vi "SavePhasor.vi"(0 "Intensity":dbl[][](array[numeric]), 1 "G Data":dbl[][](array[numeric]), 2 "S Data":dbl[][](array[numeric]), 3 "Threshold (max)":dbl=0.0035, 4 "Threshold (min)":dbl=0.002, 5 "Auto Scale?":bool=TRUE, 6 "Phasor Grids":i32, 7 "error in":errorcluster, 8 "G_max":dbl=1.1, 9 "Index Name":string, 10 "G_min":dbl=-0.1, 12 "S_max":dbl=1.1, 13 "Enable?":bool, 14 "S_min":dbl=-0.1, 15 "Time Stamp?":bool, 16 "path":path, 17 "Experiment Name":string, 18 "File Name":string, 19 "Identify Name":string, 26 "Crop Pixels":u16=40) -> (21 "img cancelled":bool, 27 "error out":errorcluster)   [LabVIEW 2018]
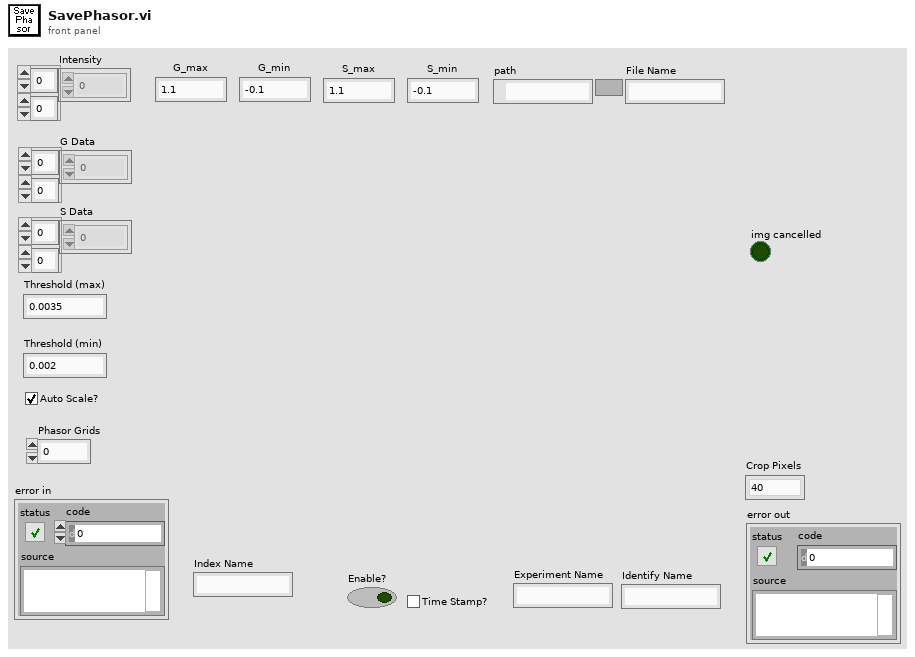
[diagram p1: front panel]
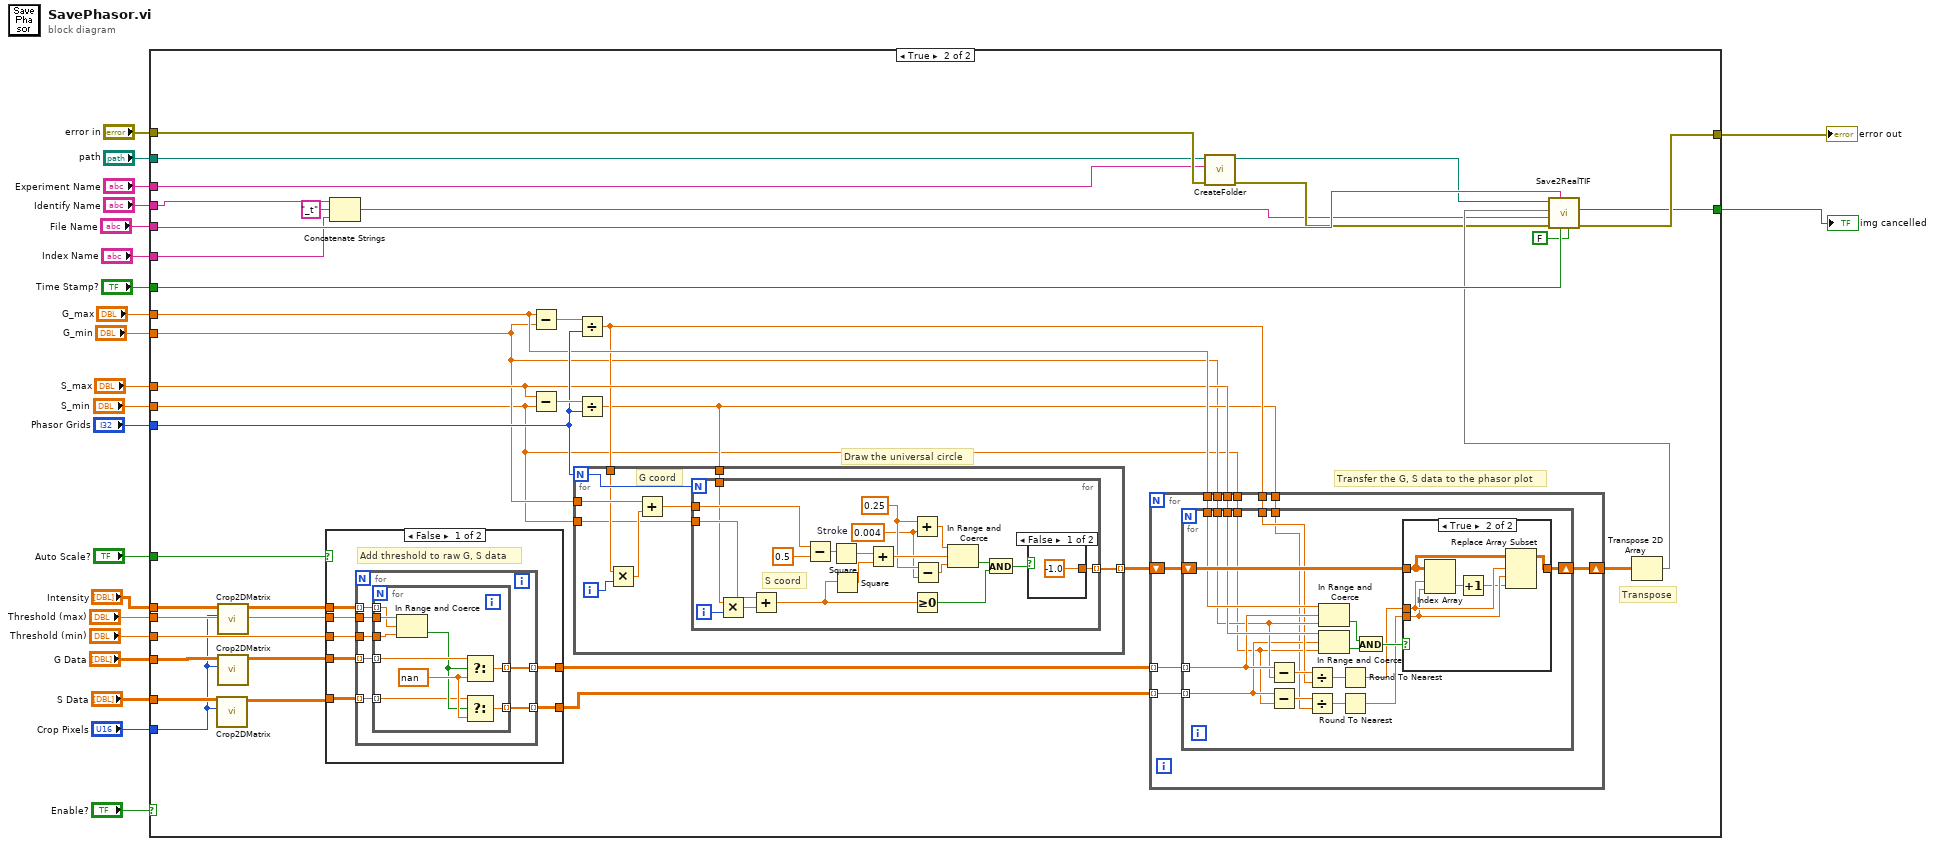
[diagram p0: block diagram]
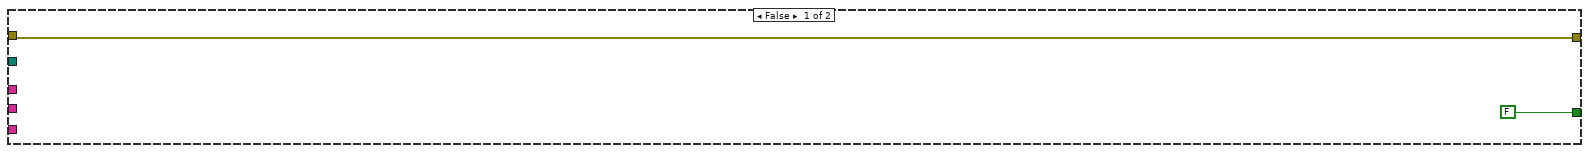
[diagram p2: hidden frame]
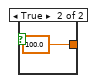
[diagram p5: hidden frame]
diagram:
  n1 = case shown="True" "Enable?" {
    tunnel: "S Data" -> [_ w37]
    tunnel: "G Data" -> [_ w38]
    tunnel: "Threshold (min)" -> [_ w59]
    tunnel: "Threshold (max)" -> [_ w58]
    tunnel: "Auto Scale?" -> [_ w57]
    tunnel: "Intensity" -> [_ w41]
    tunnel: "Phasor Grids" -> [_ w54]
    tunnel: "G_max" -> [_ w53]
    tunnel: "S_max" -> [_ w52]
    tunnel: "G_min" -> [_ w49]
    tunnel: "S_min" -> [_ w48]
    tunnel: [w24 w47] -> w11
    tunnel: "error in" -> [w24 w34]
    tunnel: [FALSE ("save cancelled") w46] -> w8
    tunnel: "path" -> [_ w33]
    tunnel: "Experiment Name" -> [_ w32]
    tunnel: "Identify Name" -> [_ w27]
    tunnel: "File Name" -> [_ w45]
    tunnel: "Time Stamp?" -> [_ w44]
    tunnel: "Crop Pixels" -> [_ w35]
    tunnel: "Index Name" -> [_ w26]
    frame False {
    }
    frame True {
      # "Transpose"
      # "Transfer the G, S data to the phasor plot"
      # "Draw the universal circle"
      n2 = call "Crop2DMatrix.vi"("Crop Pixels"=w35, "Data"=w37) -> ("Cropped Data"=w36:dbl[][])  [unwired: 9 in]
      n3 = call "Crop2DMatrix.vi"("Crop Pixels"=w35, "Data"=w41) -> ("Cropped Data"=w40:dbl[][])  [unwired: 9 in]
      n4 = call "Crop2DMatrix.vi"("Crop Pixels"=w35, "Data"=w38) -> ("Cropped Data"=w39:dbl[][])  [unwired: 9 in]
      n5 = case shown="False" w57 {
        tunnel: w40 -> [w69 _]
        tunnel: w58 -> [w68 _]
        tunnel: w59 -> [w67 _]
        tunnel: w39 -> [w66 w87]
        tunnel: w36 -> [w65 w86]
        tunnel: [w64 w87] -> w61
        tunnel: [w63 w86] -> w60
        frame False {
          # "Add threshold to raw G, S data"
          n6 = for {
            tunnel: w69 -> [w76] mode=indexing
            tunnel: w68 -> [w75]
            tunnel: [w74] -> w64 mode=indexing
            tunnel: w67 -> [w73]
            tunnel: w66 -> [w72] mode=indexing
            tunnel: w65 -> [w71] mode=indexing
            tunnel: [w70] -> w63 mode=indexing
            n7 = for {
              tunnel: w76 -> [w82] mode=indexing
              tunnel: w75 -> [w84]
              tunnel: [w85] -> w74 mode=indexing
              tunnel: w73 -> [w83]
              tunnel: w72 -> [w81] mode=indexing
              tunnel: w71 -> [w78] mode=indexing
              tunnel: [w77] -> w70 mode=indexing
              w80 = nan ("f")
              n8 = In Range and Coerce(upper limit=w84, x=w82, lower limit=w83) -> (In Range?=w79:bool)  [unwired: 1 out]
              n9 = Select(t=w81, s=w79, f=w80) -> (s? t:f=w85:dbl)
              n10 = Select(t=w78, s=w79, f=w80) -> (s? t:f=w77:dbl)
            }
          }
        }
        frame True {
        }
      }
      n11 = Concatenate Strings(w27, "_t" ("string"), w26) -> (w25:string)
      n12 = Subtract(x=w53, y=w49) -> (x-y=w56:dbl)
      n13 = Subtract(x=w52, y=w48) -> (x-y=w55:dbl)
      n14 = Divide(x=w56, y=w54) -> (x/y=w51:dbl)
      n15 = Divide(x=w55, y=w54) -> (x/y=w50:dbl)
      n16 = for {
        N: w54 -> [w132]
        tunnel: [w131] -> w62 mode=indexing
        tunnel: w49 -> [w130]
        tunnel: w51 -> [w127]
        tunnel: w48 -> [w125]
        tunnel: w50 -> [w124]
        i -> [w129]
        # "G coord"
        n17 = Multiply(x=w127, y=w129) -> (x*y=w128:dbl)
        n18 = Add(x=w130, y=w128) -> (x+y=w126:dbl)
        n19 = for {
          N: w132 -> [_]
          tunnel: w126 -> [w151]
          tunnel: [w144] -> w131 mode=indexing
          tunnel: w125 -> [w143]
          tunnel: w124 -> [w141]
          i -> [w142]
          w137 = 0.004  # Stroke
          w138 = 0.25 ("x")
          # "S coord"
          n20 = Multiply(x=w141, y=w142) -> (x*y=w140:dbl)
          n21 = Add(x=w143, y=w140) -> (x+y=w136:dbl)
          n22 = Subtract(x=w151, y=0.5) -> (x-y=w150:dbl)
          n23 = Square(x=w150) -> (x^2=w149:dbl)
          n24 = Square(x=w136) -> (x^2=w148:dbl)
          n25 = Add(x=w149, y=w148) -> (x+y=w147:dbl)
          n26 = Add(x=w138, y=w137) -> (x+y=w146:dbl)
          n27 = Greater Or Equal To 0?(x=w136) -> (x >= 0?=w133:bool)
          n28 = Subtract(x=w138, y=w137) -> (x-y=w145:dbl)
          n29 = In Range and Coerce(upper limit=w146, x=w147, lower limit=w145) -> (In Range?=w135:bool)  [unwired: 1 out]
          n30 = And(x=w135, y=w133) -> (x .and. y?=w134:bool)
          n31 = case shown="False" w134 {
            tunnel: [-1.0 ("element") 100.0 ("element")] -> w144
            frame False {
            }
            frame True {
            }
          }
        }
      }
      n32 = for {
        tunnel: w61 -> [w97] mode=indexing
        tunnel: w60 -> [w96] mode=indexing
        shift-right: [w94] -> w43
        shift-left: w62 -> [w95]
        tunnel: w53 -> [w93]
        tunnel: w49 -> [w92]
        tunnel: w52 -> [w91]
        tunnel: w48 -> [w90]
        tunnel: w51 -> [w89]
        tunnel: w50 -> [w88]
        n33 = for {
          tunnel: w97 -> [w109] mode=indexing
          tunnel: w96 -> [w103] mode=indexing
          shift-right: [w112] -> w94
          shift-left: w95 -> [w113]
          tunnel: w93 -> [w111]
          tunnel: w92 -> [w108]
          tunnel: w91 -> [w110]
          tunnel: w90 -> [w102]
          tunnel: w89 -> [w106]
          tunnel: w88 -> [w100]
          n34 = Subtract(x=w109, y=w108) -> (x-y=w107:dbl)
          n35 = Subtract(x=w103, y=w102) -> (x-y=w101:dbl)
          n36 = Divide(x=w107, y=w106) -> (x/y=w105:dbl)
          n37 = Divide(x=w101, y=w100) -> (x/y=w99:dbl)
          n38 = In Range and Coerce(upper limit=w111, x=w109, lower limit=w108) -> (In Range?=w116:bool)  [unwired: 1 out]
          n39 = In Range and Coerce(upper limit=w110, x=w103, lower limit=w102) -> (In Range?=w115:bool)  [unwired: 1 out]
          n40 = Round To Nearest(number=w105) -> (nearest integer value=w104:dbl)
          n41 = Round To Nearest(number=w99) -> (nearest integer value=w98:dbl)
          n42 = And(x=w116, y=w115) -> (x .and. y?=w114:bool)
          n43 = case shown="True" w114 {
            tunnel: w113 -> [w117 w122]
            tunnel: w104 -> [_ w121]
            tunnel: w98 -> [_ w120]
            tunnel: [w117 w118] -> w112
            frame False {
            }
            frame True {
              n44 = Index Array(array=w122, index (row)=w121, index (col)=w120) -> (element=w123:dbl)
              n45 = Increment(x=w123) -> (x+1=w119:dbl)
              n46 = Replace Array Subset(array=w122, new element=w119, index (row)=w121, index (col)=w120) -> (w118:dbl[][])
            }
          }
        }
      }
      n47 = call "CreateFolder.vi"("error in (no error)"=w34, "name"=w32, "base path"=w33) -> ("error out"=w29:errorcluster, "path out"=w30:path)  [unwired: 7 in]
      n48 = Transpose 2D Array(2D array=w43) -> (transposed array=w42:dbl[][])
      n49 = call "Save2RealTIF.vi"("Specify Range?"=FALSE ("Bound Pixel Value?"), "Time Stamp?"=w44, "File Name Prefix"=w45, "error in"=w29, "Identify Name"=w25, "Data 2D Array"=w42, "Parent Directory"=w30) -> ("error out"=w47:errorcluster, "cancelled"=w46:bool)  [unwired: 3 in]
    }
  }
  "error out" <- w11
  "img cancelled" <- w8
